vi "ExternalOutModeList.vi"(10 "List":u32) -> (2 "GetLUTModeList":cluster{string, i32})   [LabVIEW 2015]
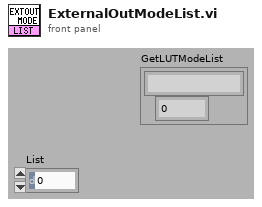
[diagram p1: front panel]
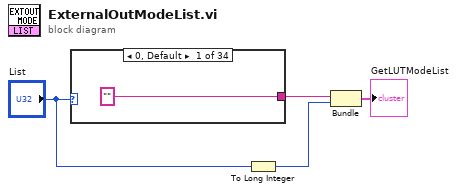
[diagram p0: block diagram]
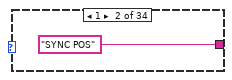
[diagram p2: hidden frame]
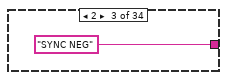
[diagram p3: hidden frame]
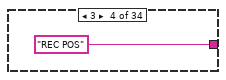
[diagram p4: hidden frame]
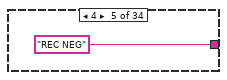
[diagram p5: hidden frame]
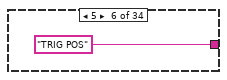
[diagram p6: hidden frame]
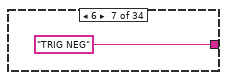
[diagram p7: hidden frame]
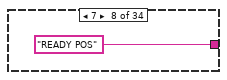
[diagram p8: hidden frame]
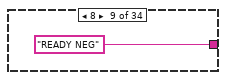
[diagram p9: hidden frame]
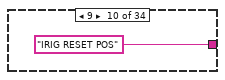
[diagram p10: hidden frame]
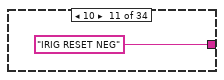
[diagram p11: hidden frame]
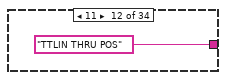
[diagram p12: hidden frame]
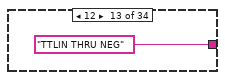
[diagram p13: hidden frame]
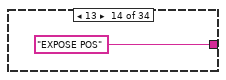
[diagram p14: hidden frame]
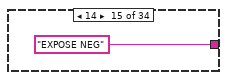
[diagram p15: hidden frame]
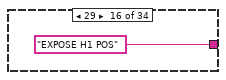
[diagram p16: hidden frame]
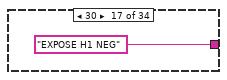
[diagram p17: hidden frame]
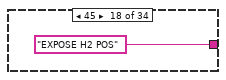
[diagram p18: hidden frame]
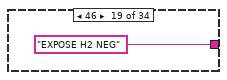
[diagram p19: hidden frame]
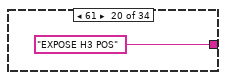
[diagram p20: hidden frame]
diagram:
  n1 = case shown="0, Default" "List" {
    tunnel: ["" "SYNC POS" "SYNC NEG" "REC POS" "REC NEG" "TRIG POS" "TRIG NEG" "READY POS" "READY NEG" "IRIG RESET POS" "IRIG RESET NEG" "TTLIN THRU POS" "TTLIN THRU NEG" "EXPOSE POS" "EXPOSE NEG" "EXPOSE H1 POS" "EXPOSE H1 NEG" "EXPOSE H2 POS" "EXPOSE H2 NEG" "EXPOSE H3 POS" "EXPOSE H3 NEG" "EXPOSE H4 POS" "EXPOSE H4 NEG" "TRIGGER" "REC POS AND SYNC POS" "REC POS AND EXPOSE POS" "ODD REC POS AND SYNC POS" "EVEN REC POS AND SYNC POS" "ODD REC POS" "EVEN REC POS" "REC START" "REC POS AND EXPOSE NEG" "STRADDLING" "REC EXPOSE"] -> w3
    frame 0, Default {
    }
    frame 1 {
    }
    frame 2 {
    }
    frame 3 {
    }
    frame 4 {
    }
    frame 5 {
    }
    frame 6 {
    }
    frame 7 {
    }
    frame 8 {
    }
    frame 9 {
    }
    frame 10 {
    }
    frame 11 {
    }
    frame 12 {
    }
    frame 13 {
    }
    frame 14 {
    }
    frame 29 {
    }
    frame 30 {
    }
    frame 45 {
    }
    frame 46 {
    }
    frame 61 {
    }
    frame 62 {
    }
    frame 77 {
    }
    frame 78 {
    }
    frame 80 {
    }
    frame 81 {
    }
    frame 82 {
    }
    frame 83 {
    }
    frame 84 {
    }
    frame 85 {
    }
    frame 86 {
    }
    frame 87 {
    }
    frame 88 {
    }
    frame 89 {
    }
    frame 90 {
    }
  }
  n2 = To Long Integer(number="List") -> (32bit integer=w2:i32)
  n3 = Bundle(w3, w2) -> (→"GetLUTModeList":cluster{string, i32})  [unwired: 1 out]
